vi "BuildEyeListFromHeader.vi"() -> ()   [LabVIEW 2022 SP3]
uses:
  <vilib>/Utility/file.llb/Read Delimited Spreadsheet (string).vi
  <vilib>/Utility/file.llb/Write Delimited Spreadsheet (string).vi
  kernel32.dll
panel:
  out "Array 2":string[](array[string])
  out "Array":string[](array[string])
  out "FloaterCount":i32
  in  "target path (use dialog)":path=path "E:/Vitreous/CUMC/Annular Array/ArrayFloatersCompiled"
  out "Floater Paths":path[](array[path])
  out "All Files in Dir":path[](array[path])
  out "All Folders":path[](array[path])
  in  "String to Append":string
  in  "Folder Path":path
  out "All Count":i32
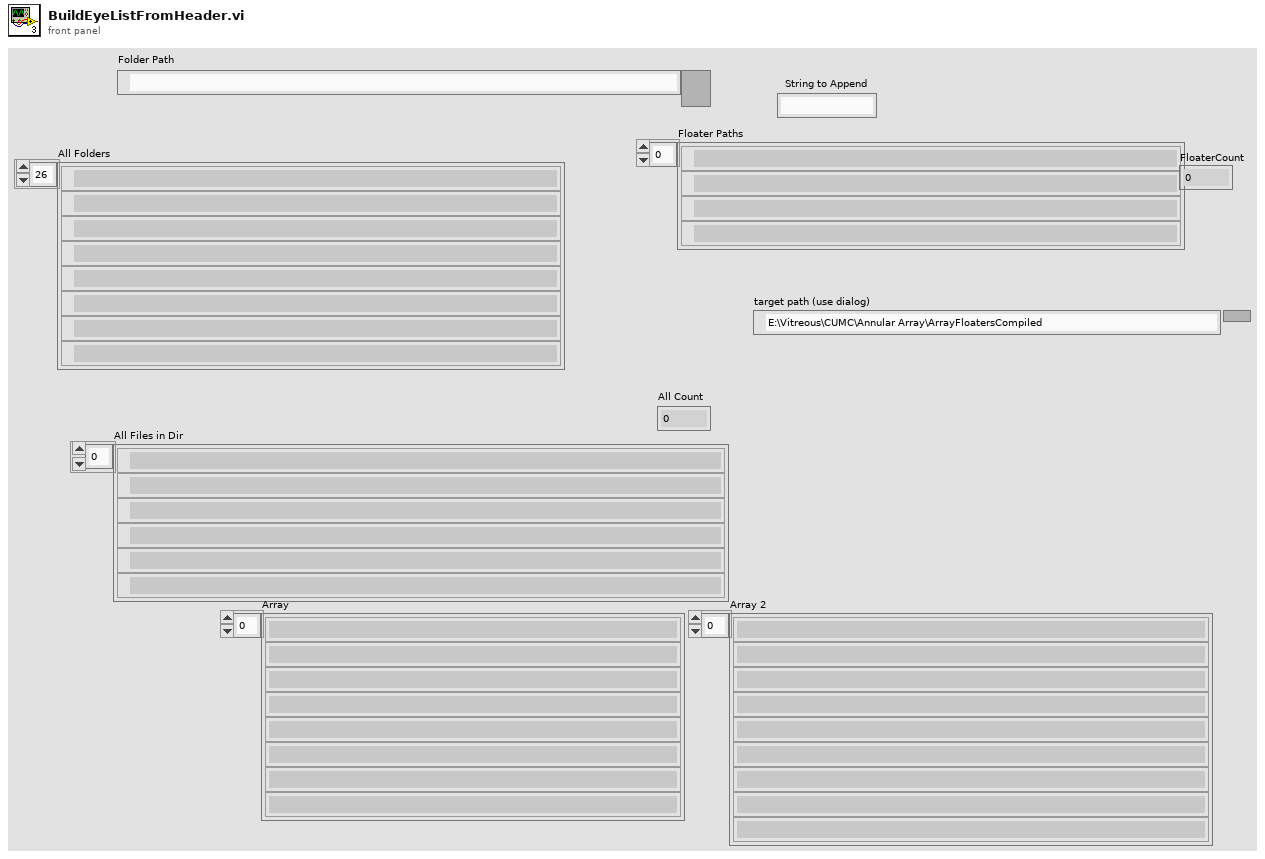
[diagram p1: front panel]
types:
  T1 = typedef "Header.ctl" = cluster{"header info":cluster{"Header":string, "Head length":i16}, "A/D info":cluster{"# rf points per line":u16, "# lines per scan":u16, "sample rate MHz":u16, "# A/D bits":i16, "# bytes per A/D":u16, "TGC Flag":u16, "A/D Type":string}, "Tranducer Info":cluster{"bandwidth":sgl, "center freq":sgl, "start freq":sgl, "ID":i32}, "Scan Info":cluster{"delay":sgl, "pivot distance":sgl, "sector scan angle":sgl, "operator":string, "Scan Mode":string, "location":string}, "Time/Date Info":cluster{"date":string, "time":string}, "RF Info":cluster{"RF file name":string, "RF file att":string, "RF cal file name":string, "RF cal file att":string}, "Patient Info":cluster{"ID":string, "extended ID":string, "age":u16, "sex":string, "previously\nscanned":string, "PSA":sgl, "LOS":u8, "Ethnicty 2":u8, "Race":u8}, "Tissue Type":cluster{"organ":i16, "disease type":i16, "disease location":i16, "IQ_pts":u16, "RcvBuffer":u8, "RcvFrame":u16, "IQBuff":u8, "IQFrame":u16, "IQPage":u8}, "Votage scaling":cluster{"Digitizer (dB)":sgl, "Gain (dB)":sgl, "Atten (dB)":sgl}, "Comment":string, "Misc Info":cluster{"avg num":u16, "c speed":i16, "Div By or SF zones":i16, "XMIT CHS":u8, "RCV CHS":u8, "Xmit angle":sgl}, "Therapy Parameters":cluster{"Theraputic Freq (MHz)":sgl, "Time on (s)":sgl, "Therapy amplitude (mV)":sgl, "Lines Before":u16, "Lines After":u16}, "Scan Settings":cluster{"Energy (uJ or V)":u8, "Damp (Ohm) or Fc":u8, "HP Filt (KHz)":u8, "LP Filt (MHz)":u8, "Gain (db)":u8, "prf (kHz)":sgl, "Distance between\nscan lines (um)":u16, "Distance between\nscan planes (um)":u16, "Scan line gap (um)":sgl, "Scan plane gap (um)":sgl}, "Compression Parameters":cluster{"F1 (MHz)":sgl, "F2 (MHz)":sgl, "% taper":sgl, "duration":sgl}, "Patient Info Xtra":cluster{"First Name":string, "Last Name":string, "Notes":string}, "ROI Box":u16[]}
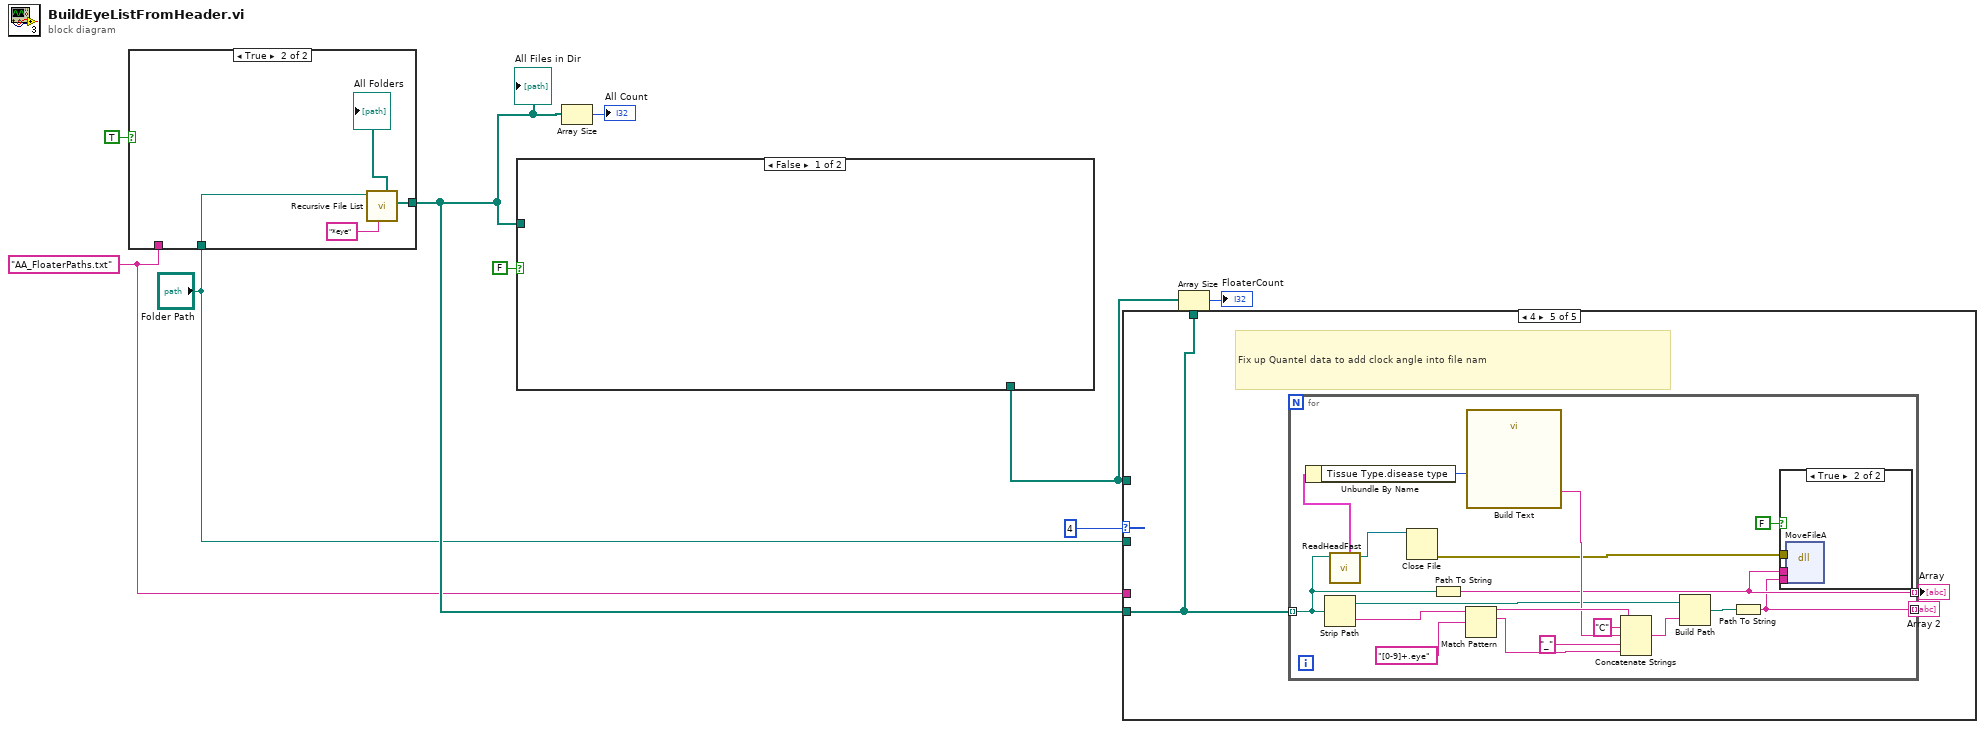
[diagram p0: block diagram]
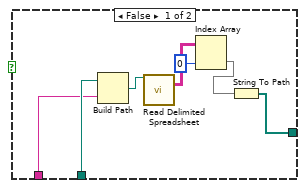
[diagram p2: hidden frame]
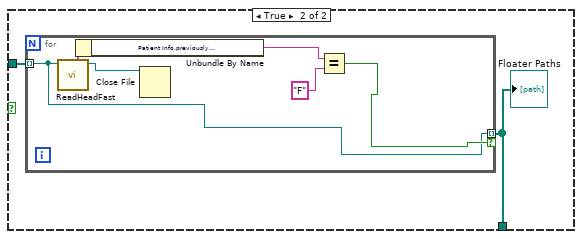
[diagram p3: hidden frame]
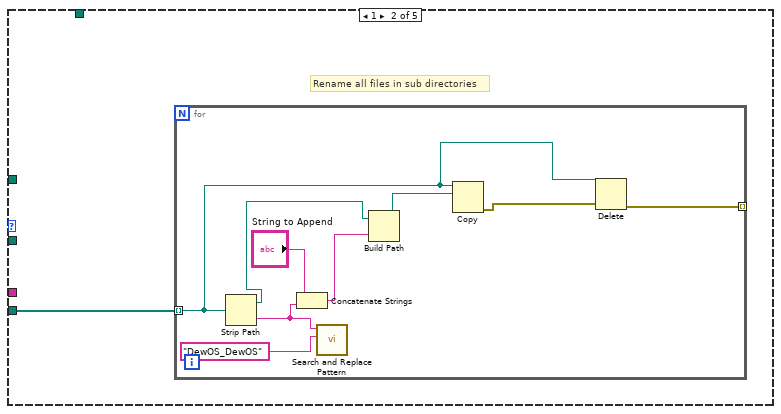
[diagram p5: hidden frame]
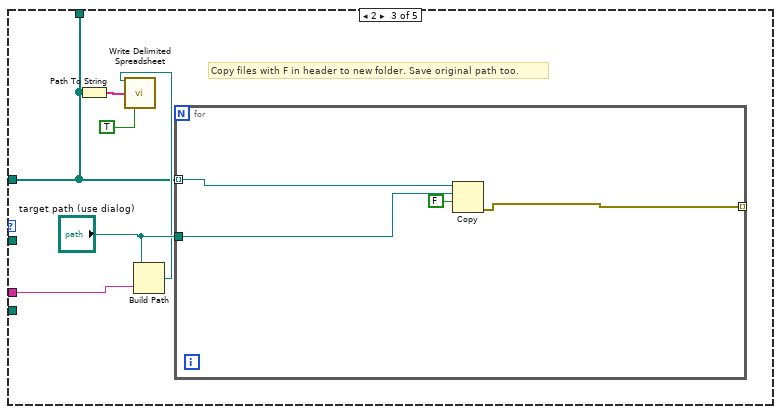
[diagram p6: hidden frame]
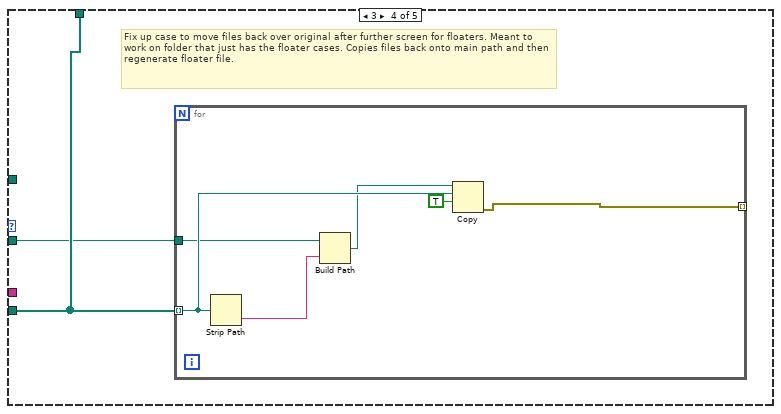
[diagram p7: hidden frame]
diagram:
  w2 = "AA_FloaterPaths.txt" ("name or relative path")
  n1 = case shown="True" TRUE {
    tunnel: [w13 w19] -> w7
    tunnel: "Folder Path" -> [w12 w18]
    tunnel: w2 -> [w11 _]
    frame False {
      n2 = Build Path(base path=w12, name or relative path=w11) -> (appended path=w10:path)
      n3 = call-poly <vilib>:"Read Delimited Spreadsheet.vi"("file path (dialog if empty)"=w10) -> ("all rows"=w16:string[][])  [unwired: 9 in, 5 out]
      n4 = Index Array(array=w16, index (col)=0 ("disabled index (col)")) -> (element=w14:string[])  [unwired: 1 in]
      n5 = String To Path(string=w14) -> (path=w13:path[])
    }
    frame True {
      n6 = call <vilib>:"Recursive File List.vi"("pattern"="*eye", "Folder Path"=w18) -> ("All Files in Dir"=w19:path[], "All Folders"=→"All Folders":path[])  [unwired: 5 in, 3 out]
    }
  }
  "All Files in Dir" <- w7
  n7 = case shown="False" FALSE {
    tunnel: w7 -> [_ w22]
    tunnel: [_ w21] -> w1
    frame False {
    }
    frame True {
      n8 = for {
        tunnel: w22 -> [w24] mode=indexing
        tunnel: [w24] -> w21 mode=indexing if=w25
        n9 = call "ReadHeadFast.vi"("new file path"=w24) -> ("refnum out"=w23:refnum<file>, "Header In"=w28:T1)  [unwired: 7 in, 2 out]
        n10 = Unbundle By Name(w28) -> ("Patient Info.previously\nscanned"=w27:string)
        n11 = Close File(refnum=w23) -> ()  [unwired: 1 in, 2 out]
        n12 = Equal?(x=w27, y="F") -> (x = y?=w25:bool)
      }
      "Floater Paths" <- w21
    }
  }
  n13 = Array Size(array=w7) -> (size(s)=→"All Count":i32)
  n14 = case shown="4" 4 ("size(s)") {
    tunnel: w7 -> [_ w29 _ w50 w59]
    tunnel: w1 -> [_ _ w40 _ _]
    tunnel: [_ _ w40 w50 w59] -> _
    tunnel: "Folder Path" -> [_ _ _ w49 _]
    tunnel: w2 -> [_ _ w39 _ _]
    frame 0, Default {
    }
    frame 1 {
      # "Rename all files in sub directories"
      n15 = for {
        tunnel: w29 -> [w34] mode=indexing
        tunnel: [w36] -> _ mode=indexing
        n16 = Strip Path(path=w34) -> (stripped path=w38:path, name=w33:string)
        n17 = Concatenate Strings("String to Append", w33) -> (w30:string)
        n18 = call <vilib>:"Search and Replace Pattern.vi"("string"=w33, "regular expression (\"\")"="DewOS_DewOS" ("String to Append")) -> ()  [unwired: 3 in, 2 out]
        n19 = Build Path(base path=w38, name or relative path=w30) -> (appended path=w37:path)
        n20 = Copy(10:w37, 11:w34) -> (0:w35:errorcluster)  [unwired: 3 in, 2 out]
        n21 = Delete(path (use dialog)=w34, error in=w35) -> (error out=w36:errorcluster)  [unwired: 3 in, 2 out]
      }
    }
    frame 2 {
      # "Copy files with F in header to new folder. Save original path too."
      n22 = Path To String(path=w40) -> (string=w44:string[])
      n23 = Build Path(base path="target path (use dialog)", name or relative path=w39) -> (appended path=w41:path)
      n24 = call-poly <vilib>:"Write Delimited Spreadsheet.vi"("file path (dialog if empty)"=w41, "1D data"=w44, "transpose? (no:F)"=TRUE ("transpose? (F)")) -> ()  [unwired: 11 in, 2 out]
      n25 = for {
        tunnel: [w45] -> _ mode=indexing
        tunnel: w40 -> [w48] mode=indexing
        tunnel: "target path (use dialog)" -> [w47]
        n26 = Copy(9:FALSE ("overwrite (F)"), 10:w47, 11:w48) -> (0:w45:errorcluster)  [unwired: 2 in, 2 out]
      }
    }
    frame 3 {
      # "Fix up case to move files back over original after further screen for floaters. Meant to work on folder that just has the floater cases. Copies files back onto main path and then regenerate floater file."
      n27 = for {
        tunnel: [w55] -> _ mode=indexing
        tunnel: w50 -> [w54] mode=indexing
        tunnel: w49 -> [w52]
        n28 = Strip Path(path=w54) -> (name=w53:string)  [unwired: 1 out]
        n29 = Build Path(base path=w52, name or relative path=w53) -> (appended path=w51:path)
        n30 = Copy(9:TRUE ("overwrite (F)"), 10:w54, 11:w51) -> (0:w55:errorcluster)  [unwired: 2 in, 2 out]
      }
    }
    frame 4 {
      # "Fix up Quantel data to add clock angle into file nam"
      n31 = for {
        tunnel: w59 -> [w66] mode=indexing
        tunnel: [w64] -> w58 mode=indexing
        tunnel: [w63] -> w57 mode=indexing
        n32 = Strip Path(path=w66) -> (stripped path=w68:path, name=w76:string)
        n33 = call "ReadHeadFast.vi"("new file path"=w66) -> ("refnum out"=w65:refnum<file>, "Header In"=w61:T1)  [unwired: 7 in, 2 out]
        n34 = Unbundle By Name(w61) -> ("Tissue Type.disease type"=w77:i16)
        n35 = Close File(refnum=w65) -> (error out=w62:errorcluster)  [unwired: 1 in, 1 out]
        n36 = Path To String(path=w66) -> (string=w64:string)
        n37 = Match Pattern(string=w76, regular expression="[0-9]+.eye") -> (before substring=w74:string, match substring=w70:string)  [unwired: 1 in, 2 out]
        n38 = call "Build Text"("d"=w77) -> ("Result"=w72:string)  [unwired: 13 in, 1 out]
        n39 = Concatenate Strings(w74, "C" ("string"), w72, "_" ("string"), w70) -> (w69:string)
        n40 = Build Path(base path=w68, name or relative path=w69) -> (appended path=w67:path)
        n41 = Path To String(path=w67) -> (string=w63:string)
        n42 = case shown="True" FALSE {
          tunnel: w64 -> [_ w80]
          tunnel: w63 -> [_ w79]
          tunnel: w62 -> [_ w78]
          frame False {
          }
          frame True {
            n43 = dll-call lib="kernel32.dll" fn="MoveFileA"(error in=w78, "arg1"=w80, "arg2"=w79) -> ()  [unwired: 5 in, 2 out]
          }
        }
      }
      "Array" <- w58
      "Array 2" <- w57
    }
  }
  n44 = Array Size(array=w1) -> (size(s)=→"FloaterCount":i32)
